vi "Color to Temperature.vi"(9 "Color":u32) -> (0 "Temperature":dbl, 3 "Slide":cluster{dbl, dbl, dbl, dbl, dbl})   [LabVIEW 2016]
uses:
  Global Flir-Ax8.vi
panel:
  out "Color":u32
  out "Closest Color Index":i32
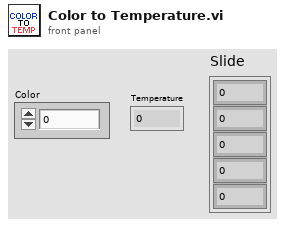
[diagram p1: front panel]
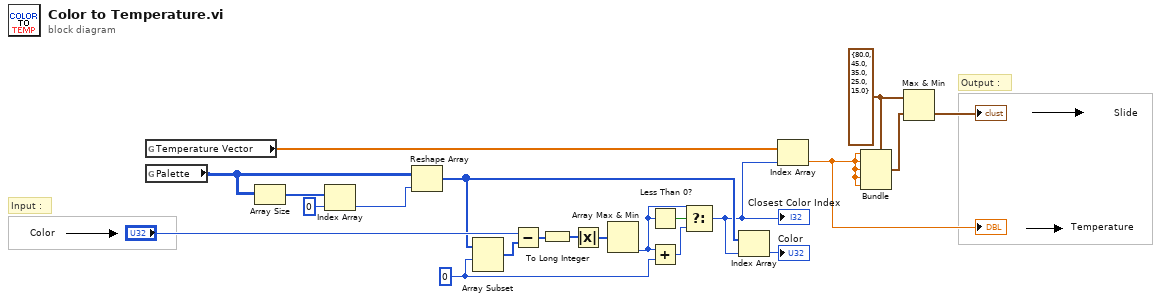
[diagram p0: block diagram]
diagram:
  w4 = cluster{dbl, dbl, dbl, dbl, dbl} {80.0, 45.0, 35.0, 25.0, 15.0} ("Slide")
  w12 = 0 ("start index (0)")
  # "Output :"
  # "Input :"
  n1 = global read "Global Flir-Ax8.vi" "Temperature Vector"() -> (w6:dbl[])
  n2 = global read "Global Flir-Ax8.vi" "Palette"() -> (w5:u32[][])
  n3 = Array Size(array=w5) -> (size(s)=w21:i32[])
  n4 = Index Array(array=w21, index=0) -> (element=w19:i32)
  n5 = Reshape Array(w5, w19) -> (w11:u32[])
  n6 = Array Subset(array=w11, index=w12) -> (w14:u32[])  [unwired: 1 in]
  n7 = Subtract(x="Color", y=w14) -> (x-y=w10:u32[])
  n8 = To Long Integer(number=w10) -> (32bit integer=w9:i32[])
  n9 = Absolute Value(x=w9) -> (abs(x)=w18:i32[])
  n10 = Array Max & Min(array=w18) -> (min index (indices)=w16:i32)  [unwired: 3 out]
  n11 = Less Than 0?(x=w16) -> (x < 0?=w17:bool)
  n12 = Add(x=w16, y=w12) -> (x+y=w15:i32)
  n13 = Select(t=w16, s=w17, f=w15) -> (s? t:f=w7:i32)
  "Closest Color Index" <- w7
  n14 = Index Array(array=w11, index=w7) -> (element=→"Color":u32)
  n15 = Index Array(array=w6, index=w7) -> (element=w1:dbl)
  "Temperature" <- w1
  n16 = Bundle(cluster=w4, w1, w1, w1, w1, w1) -> (w3:cluster{dbl, dbl, dbl, dbl, dbl})
  n17 = Max & Min(x=w4, y=w3) -> (min(x,y)=→"Slide":cluster{dbl, dbl, dbl, dbl, dbl})  [unwired: 1 out]
